vi "ttssdk.vi"(2 "Error in":errorcluster, 3 "Enter text to be spoken":string="How much wood could a woodchuck chuck if a woodchuck would chuck wood.", 4 "Choose the voice":i32(ring) items=["Microsoft Anna - English (United States)"], 5 "SpeechLib.ISpeechVoice":refnum<k7>) -> (0 "error out":errorcluster, 1 "SpeechLib.ISpeechVoice 2":refnum<k7>)   [LabVIEW 2009]
doc: "This VI is an example of Text to Speech (TTS) using the Microsoft Speech SDK 5.1. Turn off all audio applications before running this VI.\n\n1. Enter the text to be read in the text box.\n2. Choose a voice.\n3. Run the VI.\n\nNote: The first time you run this VI, the ring control might change according to the voice order that the Speech SDK installed it in. This varies on different systems. But after the first time, the ring control remains the same.\n\nFor more information on the methods and properties, refer to the documentation that is included with the SDK or visit www.microsoft.com/speech."
panel:
  out "Voices Available":string[](array[string])=["Microsoft Mike", "Microsoft Mary", "Microsoft Sam"]
  # "Select Help»Show Context Help and move the cursor over the VI icon to display help for this VI."
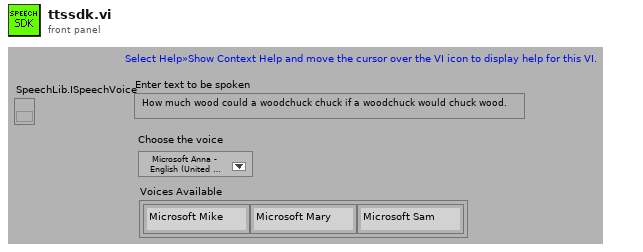
[diagram p1: front panel]
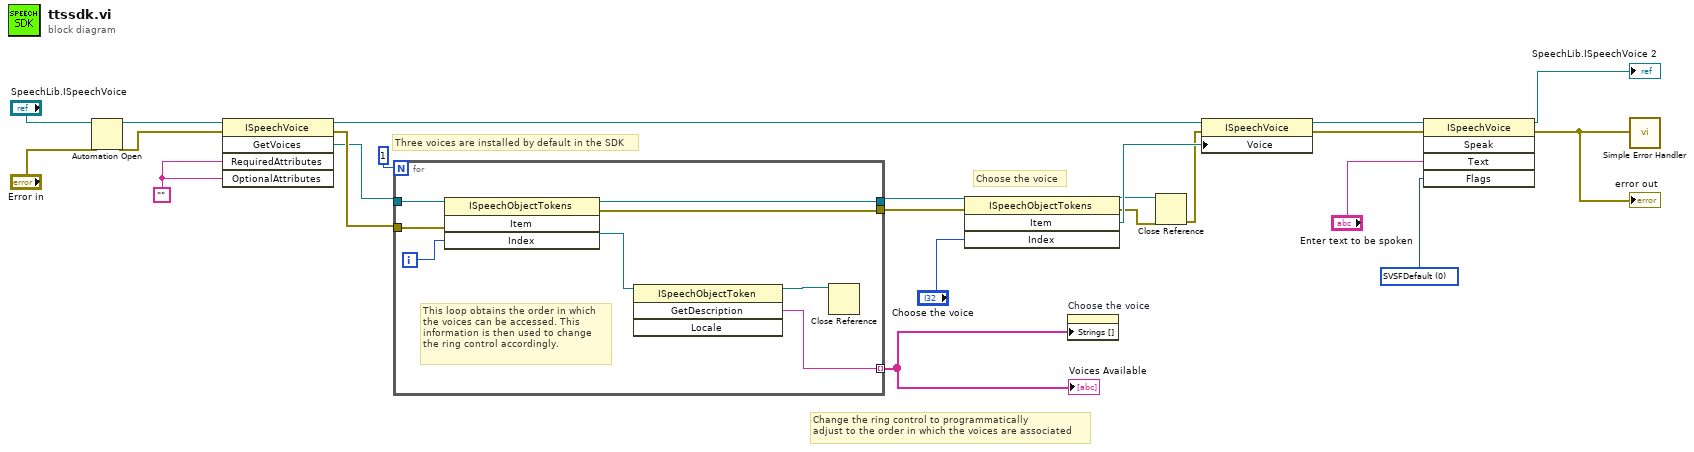
[diagram p0: block diagram]
diagram:
  w14 = ""
  w21 = 0 items=["SVSFDefault"=0, "SVSFlagsAsync"=1, "SVSFPurgeBeforeSpeak"=2, "SVSFIsFilename"=4, "SVSFIsXML"=8, "SVSFIsNotXML"=16, "SVSFPersistXML"=32, "SVSFNLPSpeakPunc, SVSFNLPMask"=64, "SVSFVoiceMask"=127, "SVSFUnusedFlags"=-128] ("Flags")
  # "Choose the voice"
  # "Three voices are installed by default in the SDK"
  # "Change the ring control to programmatically \nadjust to the order in which the voices are associated"
  n1 = Automation Open(error in (no error)="Error in", Automation Refnum="SpeechLib.ISpeechVoice") -> (Automation Refnum=w22:refnum<k7>, error out=w13:errorcluster)  [unwired: 2 in]
  n2 = invoke class="ISpeechVoice" method="GetVoices"(reference=w22, error in=w13, "RequiredAttributes"=w14, "OptionalAttributes"=w14) -> (reference out=w19:refnum<k7>, error out=w12:errorcluster, "GetVoices"=w11:refnum<k7>)  [unwired: 1 in, 2 out]
  n3 = for {
    N: 1 -> [_]
    tunnel: [w30] -> w3
    tunnel: w12 -> [w27]
    tunnel: w11 -> [w26]
    tunnel: [w25] -> w9
    tunnel: [w24] -> w8 mode=indexing
    i -> [w29]
    # "This loop obtains the order in which\nthe voices can be accessed. This \ninformation is then used to change\nthe ring control accordingly."
    n4 = invoke class="ISpeechObjectTokens" method="Item"(reference=w26, error in=w27, "Index"=w29) -> (reference out=w25:refnum<k7>, error out=w30:errorcluster, "Item"=w31:refnum<k7>)  [unwired: 1 in, 1 out]
    n5 = invoke class="ISpeechObjectToken" method="GetDescription"(reference=w31) -> (reference out=w28:refnum<k7>, "GetDescription"=w24:string)  [unwired: 3 in, 2 out]
    n6 = Close Reference(reference=w28) -> ()  [unwired: 1 in, 1 out]
  }
  "Voices Available" <- w8
  n7 = invoke class="ISpeechObjectTokens" method="Item"(reference=w9, error in=w3, "Index"="Choose the voice") -> (reference out=w5:refnum<k7>, error out=w2:errorcluster, "Item"=w15:refnum<k7>)  [unwired: 1 in, 1 out]
  n8 = property on="Choose the voice" class="Ring (strict)"("Strings []"=w8) -> ()  [unwired: 2 in, 2 out]
  n9 = Close Reference(reference=w5, error in (no error)=w2) -> (error out=w1:errorcluster)
  n10 = property class="ISpeechVoice"(reference=w19, error in=w1, "Voice"=w15) -> (reference out=w18:refnum<k7>, error out=w17:errorcluster)
  n11 = invoke class="ISpeechVoice" method="Speak"(reference=w18, error in=w17, "Text"="Enter text to be spoken", "Flags"=w21) -> (reference out=→"SpeechLib.ISpeechVoice 2":refnum<k7>, error out=w6:errorcluster)  [unwired: 1 in, 3 out]
  "error out" <- w6
  n12 = call <vilib>:"Simple Error Handler.vi"("error in (no error)"=w6) -> ()  [unwired: 4 in, 5 out]
